vi "isInRange.vi"(8 "error in (no error)":errorcluster, 10 "setup":T4, 11 "MonoCommunicator in":refnum<class "MonoCommunicator.lvclass">) -> (0 "error out":errorcluster, 2 "isInRange?":bool, 3 "MonoCommunicator out":refnum<class "MonoCommunicator.lvclass">)   [LabVIEW 2020, in "MonoCommunicator.lvclass"]
uses:
  MonoCommunicator.lvclass
  Typedefs/wavelength.ctl
  Typedefs/slitWidth.ctl
  Typedefs/GratingType.ctl
  MonoCommunicator.lvclass/MonoCommunicator.ctl
panel:
  in  "GratingType":T1=enum."Red"
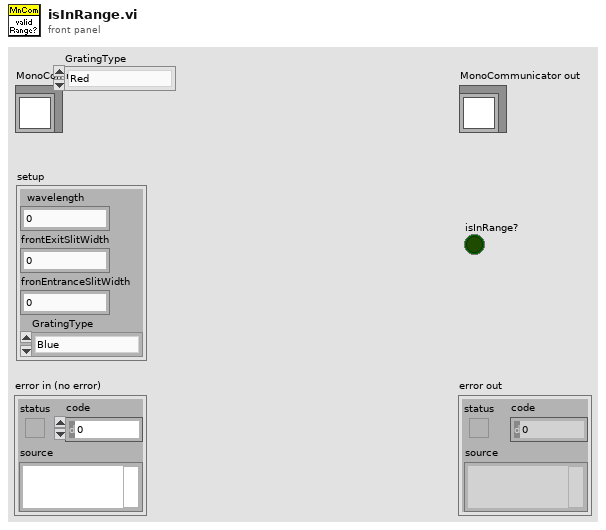
[diagram p1: front panel]
types:
  T1 = typedef "GratingType.ctl" = enum16{"Blue", "Red", "Mirror"}
  T2 = typedef "wavelength.ctl" = dbl
  T3 = typedef "slitWidth.ctl" = dbl
  T4 = cluster{"wavelength":T2, "frontExitSlitWidth":T3, "fronEntranceSlitWidth":T3, "GratingType":T1}
  T5 = typedef "Settings.lvlib/ConfigurationTypedefs.lvlib/MonochromatorSettings.ctl" = cluster{"Force Init":bool, "WavelengthMin":T2, "WavelengthMax":T2, "SlitWidthMin":T3, "SlitWidthMax":T3, "timeout":dbl}
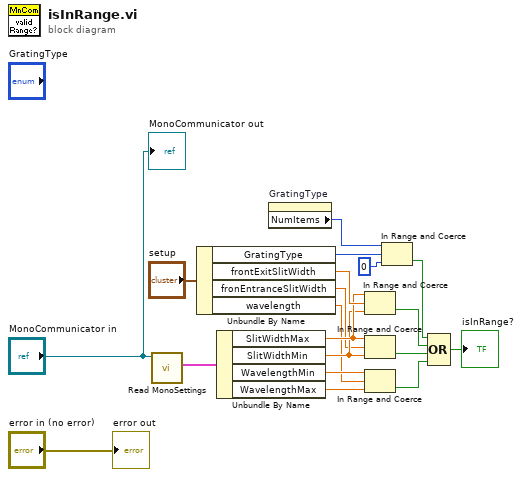
[diagram p0: block diagram]
diagram:
  n1 = call "Read MonoSettings.vi"("MonoCommunicator in"="MonoCommunicator in") -> ("MonoSettings"=w11:T5)  [unwired: 8 in, 2 out]
  n2 = Unbundle By Name("setup") -> ("GratingType"=w14:T1, "frontExitSlitWidth"=w10:T3, "fronEntranceSlitWidth"=w7:T3, "wavelength"=w4:T2)
  n3 = Unbundle By Name(w11) -> ("SlitWidthMax"=w9:T3, "SlitWidthMin"=w8:T3, "WavelengthMin"=w6:T2, "WavelengthMax"=w5:T2)
  n4 = property on="GratingType" class="Enum (strict)"() -> ("NumItems"=w18:u32)  [unwired: 2 in, 2 out]
  n5 = In Range and Coerce(upper limit=w9, x=w10, lower limit=w8) -> (In Range?=w1:bool)  [unwired: 1 out]
  n6 = In Range and Coerce(upper limit=w9, x=w7, lower limit=w8) -> (In Range?=w2:bool)  [unwired: 1 out]
  n7 = In Range and Coerce(upper limit=w6, x=w4, lower limit=w5) -> (In Range?=w3:bool)  [unwired: 1 out]
  n8 = In Range and Coerce(upper limit=w18, x=w14, lower limit=u32 0) -> (In Range?=w16:bool)  [unwired: 1 out]
  n9 = Compound Arithmetic op=OR(w16, w1, w2, w3) -> (→"isInRange?":bool)
  "error out" <- "error in (no error)"
  "MonoCommunicator out" <- "MonoCommunicator in"
